vi "drone_control.vi"() -> ()   [LabVIEW 2014]
uses:
  <vilib>/LVH/AR Drone Toolkit/Decode NavData/Typedefs/NavData Demo.ctl
  <vilib>/LVH/AR Drone Toolkit/AR Drone.lvlib
panel:
  out "NavData Out":T1
  in  "stop":bool
  in  "Control Cluster":T2 {"Yaw Speed" min=-1 max=1 step=0.01; "Vertical Speed" min=-1 max=1 step=0.01; "Pitch" min=-1 max=1 step=0.01; "Roll" min=-1 max=1 step=0.1}
  out "error out":errorcluster
  in  "Emergency Landing":bool
  in  "Takeoff/Land":bool
  in  "Hover":bool
  in  "Setup Parameters":T3={"Drone IP address"="192.168.1.1", "Home IP address"="192.168.1.2", "Flight Mode"=enum."INDOOR MODE", "Mounted Hull"=enum."INDOOR HULL", "Video Camera"=2, "Max Altitude (m)"=3.0, "Max Pitch and Roll Angle (deg)"=10.0, "Max Vertical Speed (m/s)"=0.7, "Max Yaw Speed (deg/s)"=100.0} {"Video Camera" items=["Bottom Camera"=1, "Front Camera"=0, "Front in Bottom"=3, "Bottom in Front"=2]}
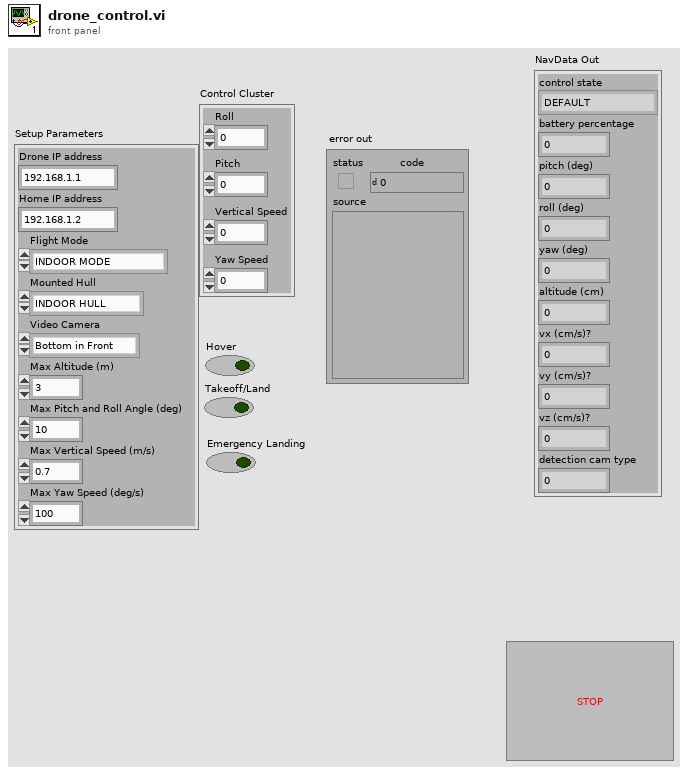
[diagram p1: front panel]
types:
  T1 = typedef "AR Drone.lvlib/NavData Demo.ctl" = cluster{"control state":enum32{"DEFAULT", "INIT", "LANDING", "FLYING", "HOVERING", "TEST", "TRANS_TAKEOFF", "TRANS_GOTOFIX", "TRANS_LANDING"}, "battery percentage":u32, "pitch (deg)":sgl, "roll (deg)":sgl, "yaw (deg)":sgl, "altitude (cm)":u32, "vx (cm/s)?":sgl, "vy (cm/s)?":sgl, "vz (cm/s)?":sgl, "detection cam type":u32}
  T2 = cluster{"Roll":sgl, "Pitch":sgl, "Vertical Speed":sgl, "Yaw Speed":sgl}
  T3 = cluster{"Drone IP address":string, "Home IP address":string, "Flight Mode":enum8{"OUTDOOR MODE", "INDOOR MODE"}, "Mounted Hull":enum8{"OUTDOOR HULL", "INDOOR HULL"}, "Video Camera":u8, "Max Altitude (m)":sgl, "Max Pitch and Roll Angle (deg)":sgl, "Max Vertical Speed (m/s)":sgl, "Max Yaw Speed (deg/s)":sgl}
  T4 = typedef "AR Drone.lvlib/AR Drone Resource.ctl" = cluster{"UDP Control Connection":refnum<k16>, "UDP NavData Connection":refnum<k16>, "UDP Video Connection (Drone 1.0)":refnum<k16>, "TCP Video Connection (Drone 2.0)":refnum<k5>, "TCP Control Port Connection":refnum<k5>, "Drone IP address":string, "Drone Command Port":u16, "Drone NavData Port":u16, "Drone Vid Stream Port":u16, "Drone TCP Control Port":u16, "Home IP address":string, "Home Command Port":u16, "Home NavData Port":u16, "Home Vid Stream Port":u16, "Drone Version":i32}
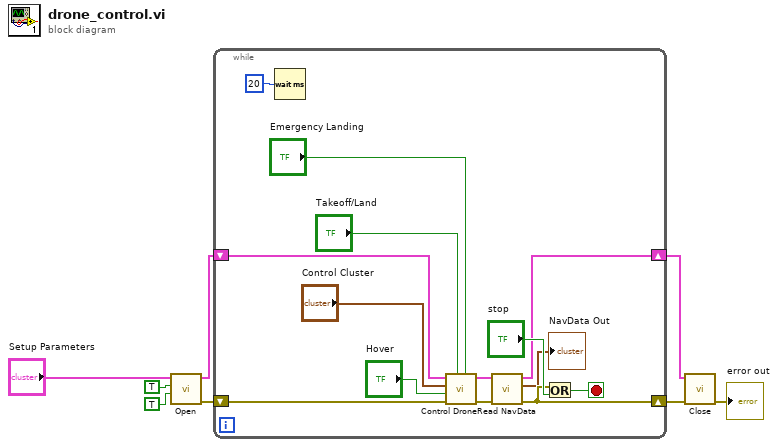
[diagram p0: block diagram]
diagram:
  n1 = call <vilib>:"Open.vi"("Init Video?"=TRUE, "Init NavData?"=TRUE, "Setup Parameters"="Setup Parameters") -> ("error out"=w1:errorcluster, "AR Drone Resource"=w2:T4)  [unwired: 7 in]
  n2 = while {
    shift-right: [w11] -> w5
    shift-left: w2 -> [w22]
    shift-right: [w10] -> w4
    shift-left: w1 -> [w21]
    stop <- w14 stop-if-true
    n3 = Wait (ms)(milliseconds to wait=u32 20) -> ()  [unwired: 1 out]
    n4 = call <vilib>:"Control Drone.vi"("Emergency Landing"="Emergency Landing", "Takeoff/Land"="Takeoff/Land", "error in (no error)"=w21, "Hover"="Hover", "Control Cluster"="Control Cluster", "AR Drone Resource"=w22) -> ("error out"=w12:errorcluster, "AR Drone Resource Out"=w13:T4)  [unwired: 4 in]
    n5 = call <vilib>:"Read NavData.vi"("error in (no error)"=w12, "AR Drone Resource"=w13) -> ("error out"=w10:errorcluster, "NavData Out"=→"NavData Out":T1, "AR Drone Resource Out"=w11:T4)  [unwired: 7 in]
    n6 = Or(x=w10, y="stop") -> (x .or. y?=w14:bool)
  }
  n7 = call <vilib>:"Close.vi"("error in (no error)"=w4, "AR Drone Resource"=w5) -> ("error out"=→"error out":errorcluster)  [unwired: 9 in]
